vi "Get Tag.vi"(8 "error in (no error)":errorcluster, 10 "ID":u32, 11 "Raw Message in":refnum<class "Raw Message.lvclass">) -> (0 "error out":errorcluster, 2 "value":refnum<class "Basic Type.lvclass">[](array[class]), 3 "Raw Message out":refnum<class "Raw Message.lvclass">)   [LabVIEW 2020, in "Protobuf RAW.lvlib" / "Raw Message.lvclass"]
uses:
  Raw Message.lvclass
  Raw Message.lvclass/Raw Message.ctl
  Tag/Basic Type.lvclass
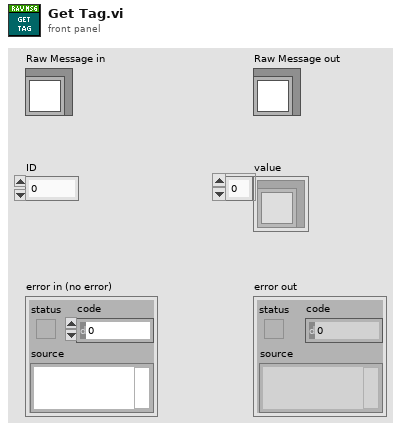
[diagram p1: front panel]
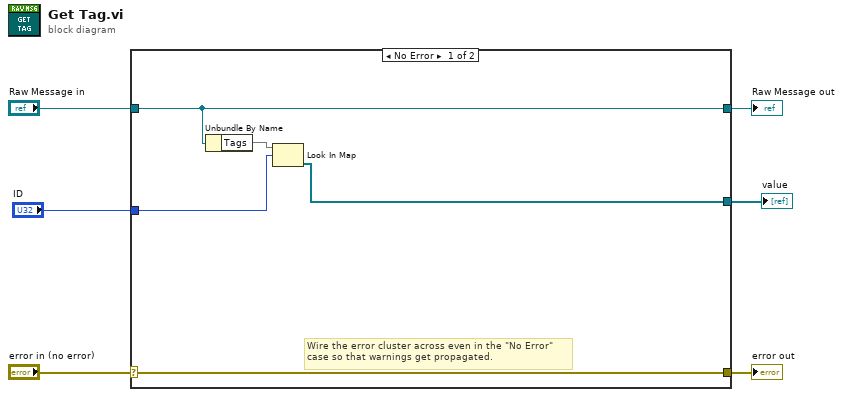
[diagram p0: block diagram]
diagram:
  n1 = case shown="No Error" "error in (no error)" {
    selector: "error in (no error)" -> [w11 w13]
    tunnel: [w11 w13] -> w5
    tunnel: [w10 w12] -> w3
    tunnel: "Raw Message in" -> [w10 w12]
    tunnel: "ID" -> [w8 _]
    tunnel: [w7 _] -> w1
    frame No Error {
      # "Wire the error cluster across even in the \"No Error\"\ncase so that warnings get propagated."
      n2 = Unbundle By Name(w10) -> ("Tags"=w9:map{u32, refnum<class "Basic Type.lvclass">[]})
      n3 = Look In Map(map=w9, key=w8) -> (value=w7:refnum<class "Basic Type.lvclass">[])  [unwired: 1 in, 1 out]
    }
    frame Error {
    }
  }
  "error out" <- w5
  "Raw Message out" <- w3
  "value" <- w1
